vi "Read From File.vi"(7 "Convert EoL? (T)":bool=TRUE, 8 "error in (no error)":errorcluster, 10 "count":i32, 11 "Text File in":refnum<class "Text File.lvclass">) -> (0 "error out":errorcluster, 2 "String":string, 3 "Text File out":refnum<class "Text File.lvclass">)   [LabVIEW 2020, in "Text File.lvclass"]
uses:
  <vilib>/gpm_packages/@cs/event-logger/Source/Text File Sink/Text File/Text File.lvclass
  <vilib>/gpm_packages/@cs/event-logger/Source/Text File Sink/Text File/Text File.lvclass/Text File.ctl
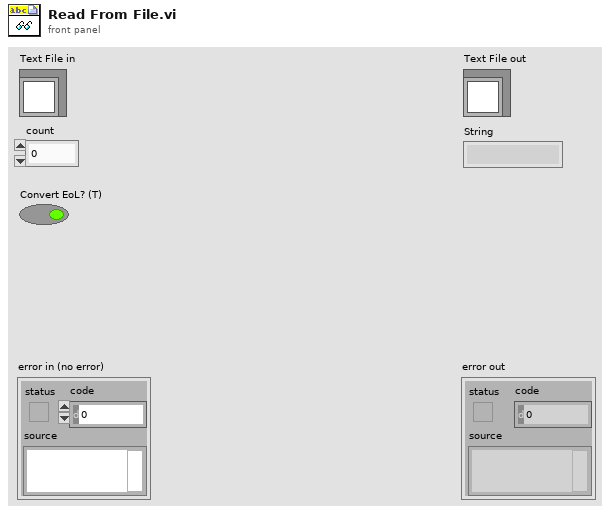
[diagram p1: front panel]
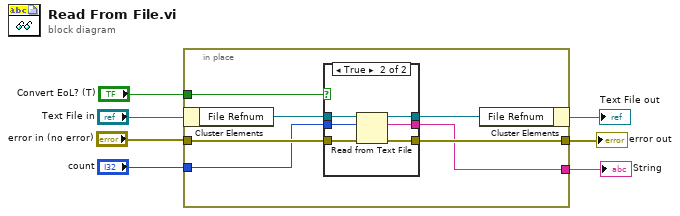
[diagram p0: block diagram]
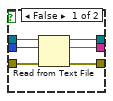
[diagram p2: hidden frame]
diagram:
  n1 = in-place {
    in-place-border: "error in (no error)" -> [w12]
    in-place-border: [w11] -> w4
    in-place-border: "count" -> [w10]
    in-place-border: [w9] -> w2
    in-place-border: "Convert EoL? (T)" -> [w8]
    n2 = in-place-cluster #1("Text File in") -> ("File Refnum"=w14:refnum<file>)
    n3 = case shown="True" w8 {
      tunnel: w14 -> [w19 w26]
      tunnel: [w16 w25] -> w13
      tunnel: w12 -> [w20 w24]
      tunnel: [w17 w23] -> w11
      tunnel: w10 -> [w18 w22]
      tunnel: [w15 w21] -> w9
      frame False {
        n4 = Read from Text File(file (use dialog)=w19, count=w18, error in=w20) -> (refnum out=w16:refnum<file>, text=w15:string, error out=w17:errorcluster)  [unwired: 1 in, 1 out]
      }
      frame True {
        n5 = Read from Text File(file (use dialog)=w26, count=w22, error in=w24) -> (refnum out=w25:refnum<file>, text=w21:string, error out=w23:errorcluster)  [unwired: 1 in, 1 out]
      }
    }
    n6 = in-place-cluster #1("File Refnum"=w13) -> (→"Text File out":refnum<class "Text File.lvclass">)
  }
  "error out" <- w4
  "String" <- w2
